vi "WSVCAP SHL Host TL Cap and DAC Table Manager.vi"(4 "Dev Mask (Add All DAC Only)":bool[](array[boolean])=[TRUE, TRUE, TRUE, TRUE, TRUE, TRUE], 5 "DUT":T1, 6 "Operation":T2=enum."Get Status", 7 "Channel (0-5)":u32, 8 "Error In":errorcluster, 10 "Voltage":dbl format="%.3f V", 11 "Data In":string[][](table)) -> (0 "Error Out":errorcluster, 3 "Table Out":string[][](table))   [LabVIEW 2017]
uses:
  Type Defs/Cap and DAC Table Manager Operation Enum.ctl
  Type Defs/WSVCAP SHL DUT Number Enum.ctl
panel:
  # "Dev 01"
  # "Dev 02"
  # "Dev 03"
  # "Dev 04"
  # "Dev 05"
  # "Dev 06"
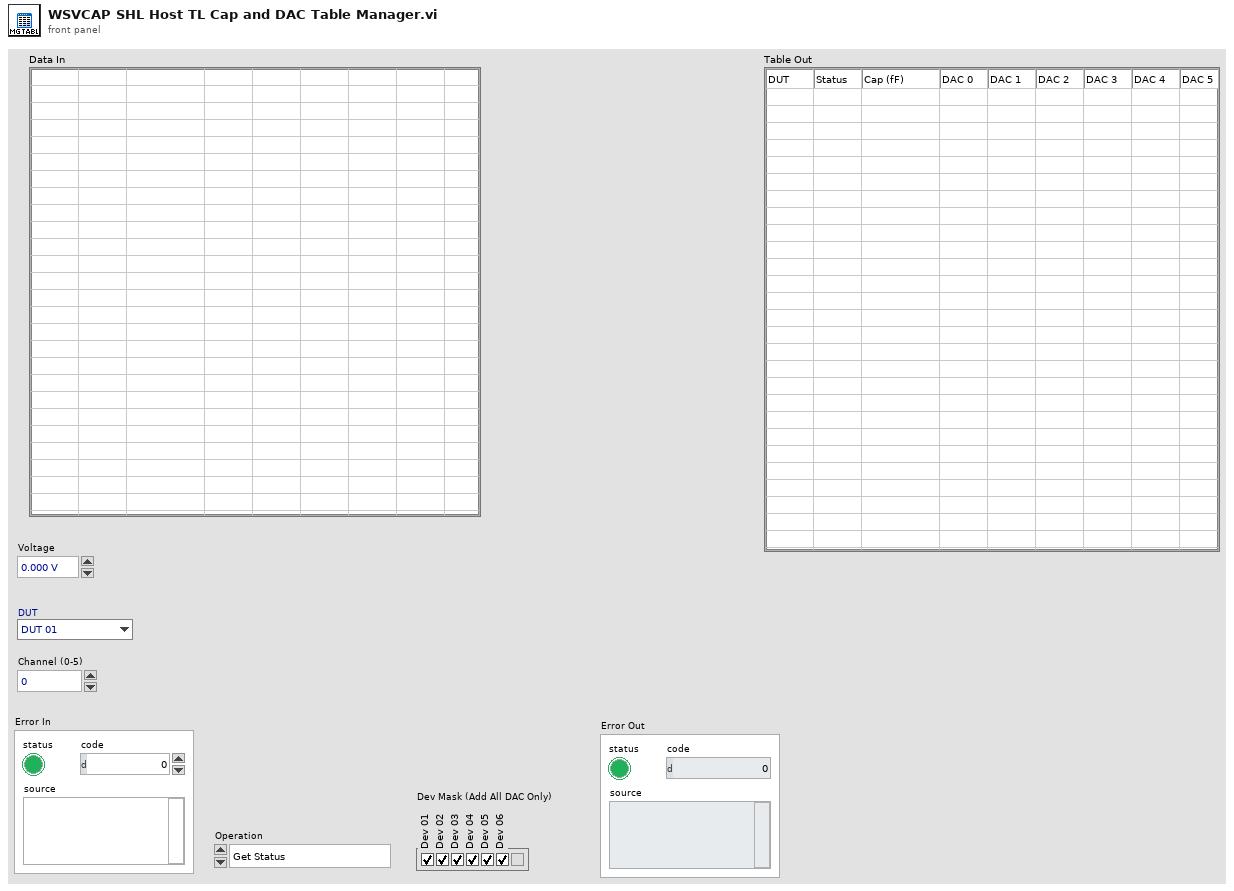
[diagram p1: front panel]
types:
  T1 = typedef "WSVCAP SHL DUT Number Enum.ctl" = enum16{"DUT 01", "DUT 02", "DUT 03", "DUT 04", "DUT 05", "DUT 06", "DUT 07", "DUT 08", "DUT 09", "DUT 10", "DUT 11", "DUT 12", "DUT 13", "DUT 14", "DUT 15", "DUT 16", "DUT 17", "DUT 18", "DUT 19", "DUT 20", "DUT 21", "DUT 22", "DUT 23", "DUT 24"}
  T2 = typedef "Cap and DAC Table Manager Operation Enum.ctl" = enum16{"Initialize", "Add Single DAC", "Add All DAC", "Add All DUT Single DAC", "Add All Cap", "Get Status"}
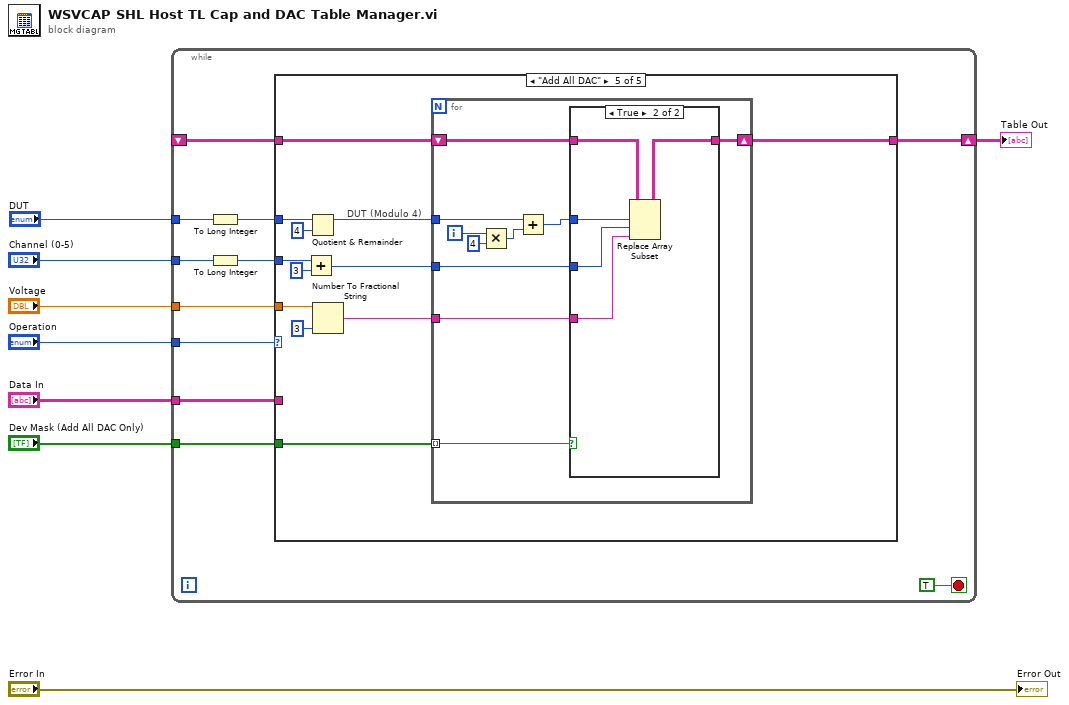
[diagram p0: block diagram]
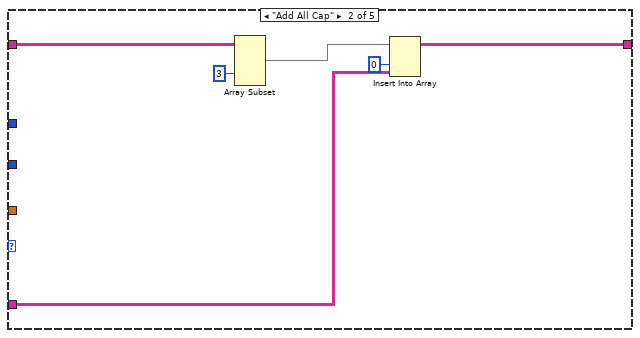
[diagram p3: hidden frame]
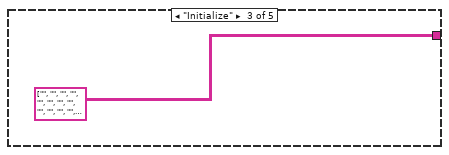
[diagram p4: hidden frame]
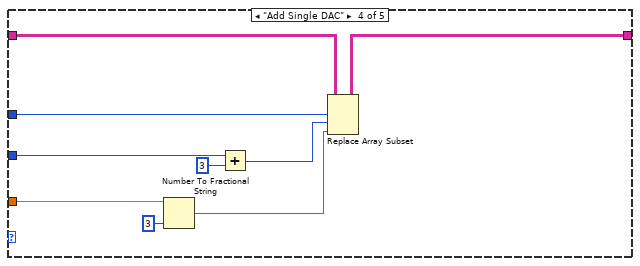
[diagram p5: hidden frame]
diagram:
  n1 = while {
    shift-right: [w18] -> w5
    shift-left: _ -> [w16]
    tunnel: "Operation" -> [w17]
    tunnel: "Data In" -> [w15]
    tunnel: "DUT" -> [w14]
    tunnel: "Channel (0-5)" -> [w12]
    tunnel: "Voltage" -> [w10]
    tunnel: "Dev Mask (Add All DAC Only)" -> [w9]
    stop <- TRUE stop-if-true
    n2 = To Long Integer(number=w14) -> (32bit integer=w13:i32)
    n3 = To Long Integer(number=w12) -> (32bit integer=w11:i32)
    n4 = case shown="\"Add All DAC\"" w17 {
      tunnel: [w20 w22 string[][] [["", "", "", "", "", "", "", "", ""], ["", "", "", "", "", "", "", "", ""], ["", "", "", "", "", "", "", "", ""], ["", "", "", "", "", "", "", "", ""], ["", "", "", "", "", "", "", "", ""], ["", "", "", "", "", "", "", "", ""], ["", "", "", "", "", "", "", "", ""], ["", "", "", "", "", "", "", "", ""], ["", "", "", "", "", "", "", "", ""], ["", "", "", "", "", "", "", "", ""], ["", "", "", "", "", "", "", "", ""], ["", "", "", "", "", "", "", "", ""], ["", "", "", "", "", "", "", "", ""], ["", "", "", "", "", "", "", "", ""], ["", "", "", "", "", "", "", "", ""], ["", "", "", "", "", "", "", "", ""], ["", "", "", "", "", "", "", "", ""], ["", "", "", "", "", "", "", "", ""], ["", "", "", "", "", "", "", "", ""], ["", "", "", "", "", "", "", "", ""], ["", "", "", "", "", "", "", "", ""], ["", "", "", "", "", "", "", "", ""], ["", "", "", "", "", "", "", "", ""], ["", "", "", "", "", "", "", "", ""]] ("Data In") w35 w47] -> w18
      tunnel: w16 -> [w20 w21 _ w36 w48]
      tunnel: w15 -> [_ w23 _ _ _]
      tunnel: w13 -> [_ _ _ w34 w40]
      tunnel: w11 -> [_ _ _ w33 w46]
      tunnel: w10 -> [_ _ _ w32 w45]
      tunnel: w9 -> [_ _ _ _ w37]
      frame Default {
      }
      frame "Add All Cap" {
        n5 = Array Subset(array=w21, index (col)=3 ("index")) -> (w25:string[][])  [unwired: 3 in]
        n6 = Insert Into Array(array=w25, index (col)=0 ("disabled index (col)"), new element=w23) -> (w22:string[][])  [unwired: 1 in]
      }
      frame "Initialize" {
      }
      frame "Add Single DAC" {
        n7 = Number To Fractional String(number=w32, precision (6)=i16 3) -> (F-format string=w30:string)  [unwired: 2 in]
        n8 = Add(x=w33, y=3) -> (x+y=w29:i32)
        n9 = Replace Array Subset(array=w36, new element=w30, index (row)=w34, index (col)=w29) -> (w35:string[][])
      }
      frame "Add All DAC" {
        # "DUT (Modulo 4)"
        n10 = Add(x=w46, y=3) -> (x+y=w42:i32)
        n11 = Quotient & Remainder(x=w40, y=4) -> (x-y*floor(x/y)=w38:i32)  [unwired: 1 out]
        n12 = Number To Fractional String(number=w45, precision (6)=i16 3) -> (F-format string=w43:string)  [unwired: 2 in]
        n13 = for {
          tunnel: w43 -> [w56]
          tunnel: w42 -> [w55]
          tunnel: w38 -> [w53]
          shift-right: [w57] -> w47
          shift-left: w48 -> [w58]
          tunnel: w37 -> [w54] mode=indexing
          i -> [w52]
          n14 = Multiply(x=w52, y=4) -> (x*y=w50:i32)
          n15 = Add(x=w53, y=w50) -> (x+y=w49:i32)
          n16 = case shown="True" w54 {
            tunnel: w58 -> [w59 w64]
            tunnel: [w59 w63] -> w57
            tunnel: w56 -> [_ w62]
            tunnel: w55 -> [_ w61]
            tunnel: w49 -> [_ w60]
            frame False {
            }
            frame True {
              n17 = Replace Array Subset(array=w64, new element=w62, index (row)=w60, index (col)=w61) -> (w63:string[][])
            }
          }
        }
      }
    }
  }
  "Table Out" <- w5
  "Error Out" <- "Error In"
